vi "Apply Stimulus Property.vi"(0 "State in":refnum<class "State.lvclass">, 5 "chan":string, 7 "param":string, 9 "value":dbl, 11 "error in (no error)":errorcluster) -> (4 "State out":refnum<class "State.lvclass">, 15 "error out":errorcluster)   [LabVIEW 2020, in "State.lvclass"]
uses:
  State.lvclass
  State.lvclass/State.ctl
  epl-vi-lib/Signal Synthesis VIs/4th Generation/Classes/SignalManager/SignalManager.lvclass
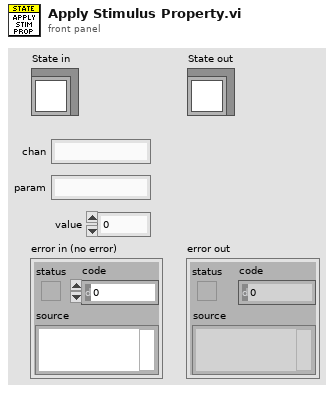
[diagram p1: front panel]
types:
  T1 = typedef "Tosca-Grating.ctl" = cluster{"Type":T2, "Orientation (deg)":dbl, "Spatial frequency (cpd)":dbl, "Velocity (Hz)":dbl, "Contrast":dbl, "Background intensity":dbl, "Duration (ms)":dbl, "Phase (cycles)":dbl}
  T2 = typedef "Tosca-Grating Type.ctl" = enum16{"OFF", "Square", "Sine"}
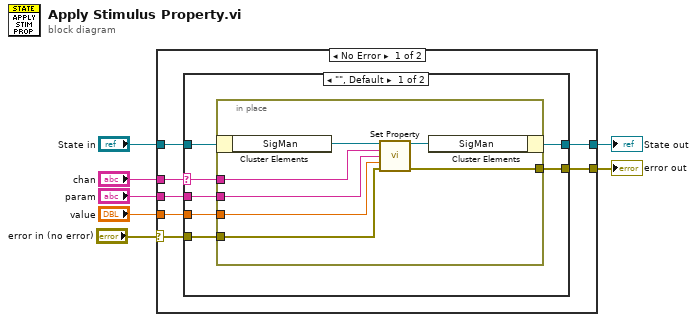
[diagram p0: block diagram]
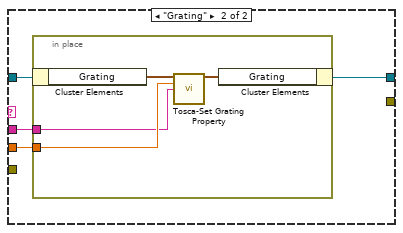
[diagram p2: hidden frame]
diagram:
  n1 = case shown="No Error" "error in (no error)" {
    selector: "error in (no error)" -> [w9 w38]
    tunnel: [w8 w38] -> w1
    tunnel: [w13 w37] -> w5
    tunnel: "State in" -> [w14 w37]
    tunnel: "chan" -> [w12 _]
    tunnel: "param" -> [w11 _]
    tunnel: "value" -> [w10 _]
    frame No Error {
      n2 = case shown="\"\", Default" w12 {
        selector: w12 -> [w19 _]
        tunnel: w14 -> [w21 w32]
        tunnel: [w20 w29] -> w13
        tunnel: w11 -> [w18 w30]
        tunnel: w10 -> [w17 w31]
        tunnel: w9 -> [w16 _]
        tunnel: [w15 _] -> w8
        frame "", Default {
          n3 = in-place {
            in-place-border: w19 -> [w26]
            in-place-border: w18 -> [w25]
            in-place-border: w17 -> [w24]
            in-place-border: w16 -> [w23]
            in-place-border: [w22] -> w15
            n4 = in-place-cluster #1(w21) -> ("SigMan"=w28:refnum<class "SignalManager.lvclass">)
            n5 = call "Set Property.vi"("SigMan in"=w28, "chan"=w26, "param"=w25, "value"=w24, "error in (no error)"=w23) -> ("SigMan out"=w27:refnum<class "SignalManager.lvclass">, "error out"=w22:errorcluster)  [unwired: 9 in]
            n6 = in-place-cluster #1("SigMan"=w27) -> (w20:refnum<class "State.lvclass">)
          }
        }
        frame "Grating" {
          n7 = in-place {
            in-place-border: w31 -> [w34]
            in-place-border: w30 -> [w33]
            n8 = in-place-cluster #2(w32) -> ("Grating"=w36:T1)
            n9 = call "Tosca-Set Grating Property.vi"("Grating in"=w36, "value"=w34, "property"=w33) -> ("Grating out"=w35:T1)  [unwired: 12 in]
            n10 = in-place-cluster #2("Grating"=w35) -> (w29:refnum<class "State.lvclass">)
          }
        }
      }
    }
    frame Error {
    }
  }
  "error out" <- w1
  "State out" <- w5
